vi "GLOBAL CENTER FREQ ENABLE.vi"(6 "READ ONLY (T)":bool, 8 "error in":errorcluster {"code" format="%.0x"}, 10 "ON/OFF":string(combo)="ALL", 11 "Session In":refnum<visa-resource-name>="GPIB0::18::INSTR") -> (0 "error out":errorcluster {"code" format="%.0x"}, 2 "READ":string, 3 "Session Out":refnum<visa-resource-name>)   [LabVIEW 2018]
uses:
  Agilent MXA Series/Agilent MXA Series.lvlib
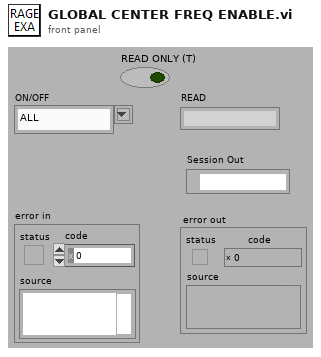
[diagram p1: front panel]
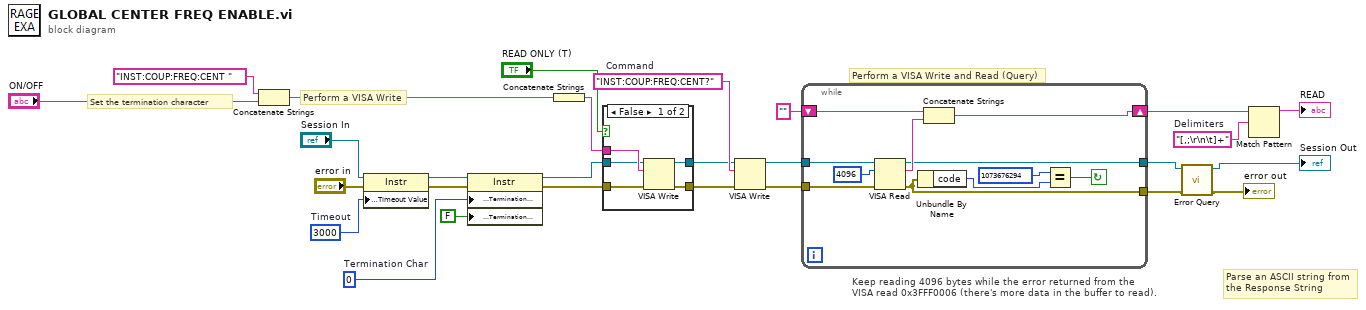
[diagram p0: block diagram]
diagram:
  w9 = "[,;\r\n\t]+"  # Delimiters
  w11 = "INST:COUP:FREQ:CENT?"  # Command
  w22 = u8 0  # Termination Char
  w26 = u32 3000  # Timeout
  # "Parse an ASCII string from the Response String"
  # "Perform a VISA Write and Read (Query)"
  # "Keep reading 4096 bytes while the error returned from the\nVISA read 0x3FFF0006 (there's more data in the buffer to read)."
  # "Perform a VISA Write"
  # "Set the termination character"
  n1 = Concatenate Strings("INST:COUP:FREQ:CENT " ("staticText"), "ON/OFF") -> (w15:string)
  n2 = property class="Instr"(reference="Session In", error in="error in", "General Settings:Timeout Value"=w26) -> (reference out=w21:refnum<visa-resource-name>, error out=w24:errorcluster)
  n3 = property class="Instr"(reference=w21, error in=w24, "Message Based Settings:Termination Character"=w22, "Message Based Settings:Termination Character Enable"=FALSE ("enable")) -> (reference out=w7:refnum<visa-resource-name>, error out=w23:errorcluster)
  n4 = Concatenate Strings(w15) -> (w16:string)
  n5 = case shown="False" "READ ONLY (T)" {
    tunnel: w23 -> [w32 w33]
    tunnel: [w31 w33] -> w17
    tunnel: w16 -> [w30 _]
    tunnel: w7 -> [w29 w34]
    tunnel: [w28 w34] -> w6
    frame False {
      n6 = VISA Write(VISA resource name=w29, write buffer=w30, error in (no error)=w32) -> (VISA resource name out=w28:refnum<visa-resource-name>, error out=w31:errorcluster)  [unwired: 1 out]
    }
    frame True {
    }
  }
  n7 = VISA Write(VISA resource name=w6, write buffer=w11, error in (no error)=w17) -> (VISA resource name out=w14:refnum<visa-resource-name>, error out=w13:errorcluster)  [unwired: 1 out]
  n8 = while {
    tunnel: w14 -> [w42]
    shift-right: [w36] -> w8
    shift-left: "" -> [w41]
    tunnel: w13 -> [w39]
    tunnel: [w38] -> w2
    tunnel: [w35] -> w4
    stop <- w37 continue-if-true
    n9 = VISA Read(VISA resource name=w42, byte count=u32 4096 ("byte count (0)"), error in (no error)=w39) -> (VISA resource name out=w35:refnum<visa-resource-name>, read buffer=w40:string, error out=w38:errorcluster)  [unwired: 1 out]
    n10 = Unbundle By Name(w38) -> ("code"=w44:i32)
    n11 = Concatenate Strings(w41, w40) -> (w36:string)
    n12 = Equal?(x=1073676294, y=w44) -> (x = y?=w37:bool)
  }
  n13 = call "Error Query.vi"("error in (no error)"=w2, "VISA resource name"=w4) -> ("error out"=→"error out":errorcluster, "VISA resource name out"=→"Session Out":refnum<visa-resource-name>)  [unwired: 6 in, 2 out]
  n14 = Match Pattern(string=w8, regular expression=w9) -> (before substring=→"READ":string)  [unwired: 4 out]
